vi "Check if Nests Destroyed.vi"(11 "Self Actor":refnum<class "Self Actor.lvclass">) -> (2 "Nest Actors Destroyed?":bool)   [LabVIEW 2021, in "LVCAM.lvlib" / "Self Actor.lvclass"]
uses:
  Self Actor.lvclass
  Self Actor.lvclass/Self Actor.ctl
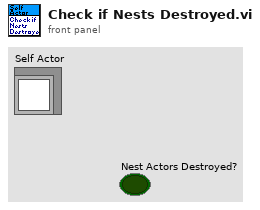
[diagram p1: front panel]
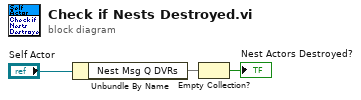
[diagram p0: block diagram]
diagram:
  n1 = Unbundle By Name("Self Actor") -> ("Nest Msg Q DVRs"=w1:set{refnum<data-value>})
  n2 = Empty Collection?(1:w1) -> (0:→"Nest Actors Destroyed?":bool)
